vi "Reflux On Batch.vi"() -> ()   [LabVIEW 2017]
panel:
  in  "Reflux On":bool
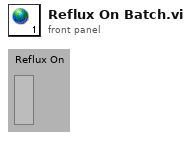
[diagram p1: front panel]
diagram:
